vi "(SubVI)Scope_Graph_Array Subset.vi"(10 "length":i32, 11 "data in":dbl[][](array[numeric])) -> (3 "data out":dbl[][](array[numeric]), 5 "enough":bool)   [LabVIEW 2020]
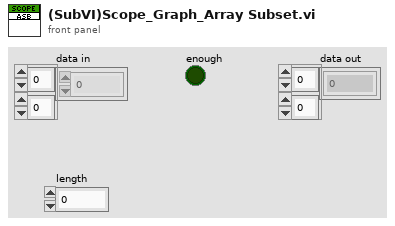
[diagram p1: front panel]
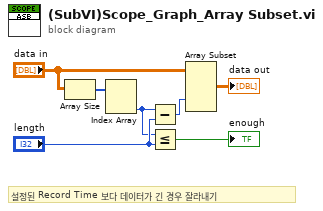
[diagram p0: block diagram]
diagram:
  # "설정된 Record Time 보다 데이터가 긴 경우 잘라내기"
  n1 = Array Size(array="data in") -> (size(s)=w4:i32[])
  n2 = Index Array(array=w4) -> (element #2=w2:i32)  [unwired: 2 in, 1 out]
  n3 = Subtract(x=w2, y="length") -> (x-y=w6:i32)
  n4 = Less Or Equal?(x=w2, y="length") -> (x <= y?=→"enough":bool)
  n5 = Array Subset(array="data in", index (col)=w6) -> (→"data out":dbl[][])  [unwired: 3 in]
